vi "Trace UI Message.vi"(7 "Position":T1[](array[typedef]), 9 "Command":string, 10 "SweepProperties":T3) -> (1 "UI Msg String":string)   [LabVIEW 2018]
uses:
  Datalog/DatalogSubvis/SearchableTag.ctl
  RF Direction.ctl
  PolarizationSelect.ctl
  APARMainSubvis/VXM Public API/singleAxisMoveDef.ctl
  APARMainSubvis/VXM Public API/mmWaveAxis.ctl
  Datalog/DataLog.lvclass
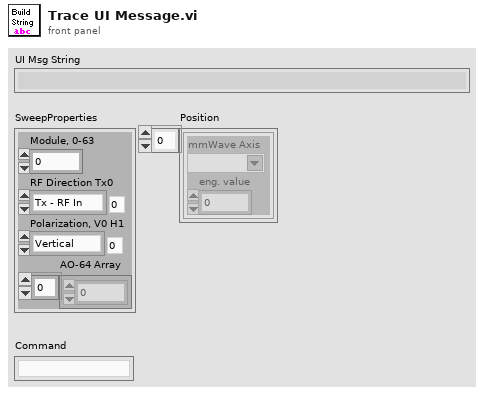
[diagram p1: front panel]
types:
  T1 = typedef "singleAxisMoveDef.ctl" = cluster{"mmWave Axis":T2, "eng. value":dbl}
  T2 = typedef "mmWaveAxis.ctl" = string
  T3 = typedef "DataLog.lvclass/SearchableTag.ctl" = cluster{"Module, 0-63":i32, "RF Direction Tx0":T4, "Polarization, V0 H1":T5, "AO-64 Array":dbl[]}
  T4 = typedef "RF Direction.ctl" = enum16{"Tx - RF In", "Rx - RF Out"}
  T5 = typedef "PolarizationSelect.ctl" = enum16{"Vertical", "Horizontal"}
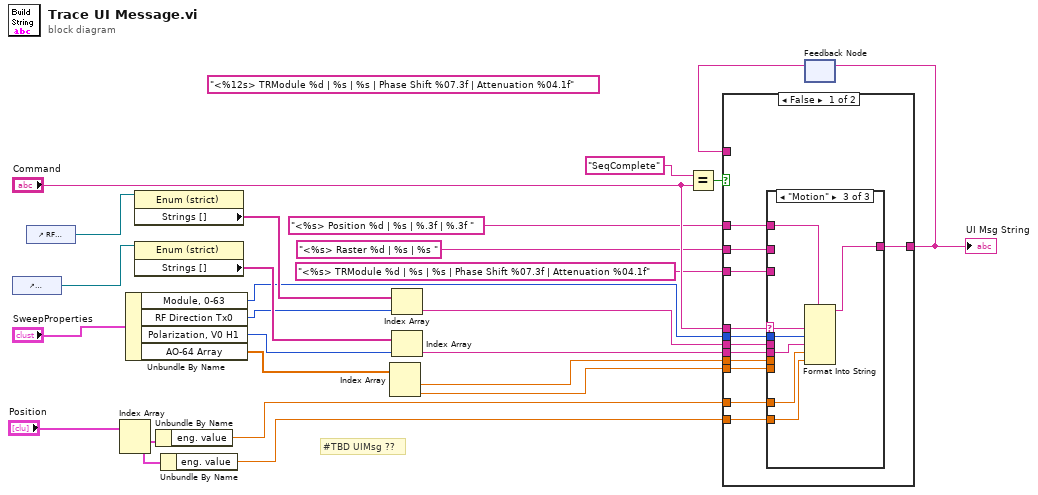
[diagram p0: block diagram]
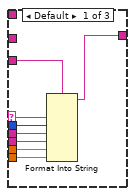
[diagram p2: hidden frame]
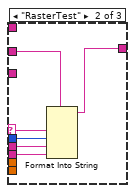
[diagram p3: hidden frame]
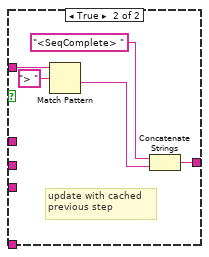
[diagram p4: hidden frame]
diagram:
  (unwired) "<%12s> TRModule %d | %s | %s | Phase Shift %07.3f | Attenuation %04.1f" ("format string")
  # "#TBD UIMsg ??"
  n1 = control-ref of="Polarization, V0 H1"() -> (w25:refnum<vi>)
  n2 = control-ref of="RF Direction Tx0"() -> (w21:refnum<vi>)
  n3 = Index Array(array="Position") -> (element #1=w4:T1, element #2=w3:T1)  [unwired: 2 in]
  n4 = Unbundle By Name("SweepProperties") -> ("Module, 0-63"=w19:i32, "RF Direction Tx0"=w20:T4, "Polarization, V0 H1"=w23:T5, "AO-64 Array"=w8:dbl[])
  n5 = property class="Enum (strict)"(reference=w21) -> ("Strings []"=w22:string[])  [unwired: 1 in, 2 out]
  n6 = property class="Enum (strict)"(reference=w25) -> ("Strings []"=w24:string[])  [unwired: 1 in, 2 out]
  n7 = Unbundle By Name(w4) -> ("eng. value"=w2:dbl)
  n8 = Unbundle By Name(w3) -> ("eng. value"=w1:dbl)
  n9 = Index Array(array=w8) -> (element #1=w7:dbl, element #2=w6:dbl)  [unwired: 2 in]
  n10 = Index Array(array=w22, index=w20) -> (element=w18:string)
  n11 = Index Array(array=w24, index=w23) -> (element=w17:string)
  n12 = Equal?(x="SeqComplete", y="Command") -> (x = y?=w13:bool)
  n13 = feedback #1() -> (w12:string)  [unwired: 1 in]
  n14 = case shown="False" w13 {
    tunnel: "<%s> TRModule %d | %s | %s | Phase Shift %07.3f | Attenuation %04.1f" ("format string") -> [w38 _]
    tunnel: w19 -> [w37 _]
    tunnel: w7 -> [w36 _]
    tunnel: w6 -> [w35 _]
    tunnel: w18 -> [w34 _]
    tunnel: w17 -> [w33 _]
    tunnel: "Command" -> [w31 _]
    tunnel: [w32 w62] -> w14
    tunnel: w12 -> [_ w63]
    tunnel: "<%s> Raster %d | %s | %s " ("format string") -> [w30 _]
    tunnel: "<%s> Position %d | %s | %.3f | %.3f " ("format string") -> [w29 _]
    tunnel: w2 -> [w28 _]
    tunnel: w1 -> [w27 _]
    frame False {
      n15 = case shown="\"Motion\"" w31 {
        selector: w31 -> [w39 w48 w57]
        tunnel: w38 -> [w46 _ _]
        tunnel: w37 -> [w45 w52 w59]
        tunnel: w36 -> [w44 _ _]
        tunnel: w35 -> [w43 _ _]
        tunnel: w34 -> [w42 w51 _]
        tunnel: w33 -> [w41 w50 w55]
        tunnel: [w40 w49 w58] -> w32
        tunnel: w30 -> [_ w47 _]
        tunnel: w29 -> [_ _ w56]
        tunnel: w28 -> [_ _ w54]
        tunnel: w27 -> [_ _ w53]
        frame Default {
          n16 = Format Into String(format string=w46, w39, w45, w42, w41, w44, w43) -> (resulting string=w40:string)  [unwired: 2 in, 1 out]
        }
        frame "RasterTest" {
          n17 = Format Into String(format string=w47, w48, w52, w51, w50) -> (resulting string=w49:string)  [unwired: 2 in, 1 out]
        }
        frame "Motion" {
          n18 = Format Into String(format string=w56, w57, w59, w55, w54, w53) -> (resulting string=w58:string)  [unwired: 2 in, 1 out]
        }
      }
    }
    frame True {
      # "update with cached \nprevious step"
      n19 = Match Pattern(string=w63, regular expression="> ") -> (after substring=w60:string)  [unwired: 1 in, 3 out]
      n20 = Concatenate Strings("<SeqComplete> ", w60) -> (w62:string)
    }
  }
  "UI Msg String" <- w14
  n21 = feedback-in #1(w14) -> ()
